vi "Init.vi"(8 "error in (no error)":errorcluster, 11 "Data in":refnum<class "SynchType_DBL.lvclass">) -> (0 "error out":errorcluster, 3 "Data out":refnum<class "SynchType_DBL.lvclass">)   [LabVIEW 2021, in "BT.lvlib" / "SynchType_DBL.lvclass"]
doc: "Abstract Data Classes 2.1.1.12\nTim Streeter - TSA\nCopyright (c) 2024, TSA"
uses:
  SynchType_DBL.lvclass
  SynchType_DBL.lvclass/SynchType_DBL.ctl
  Type.ctl
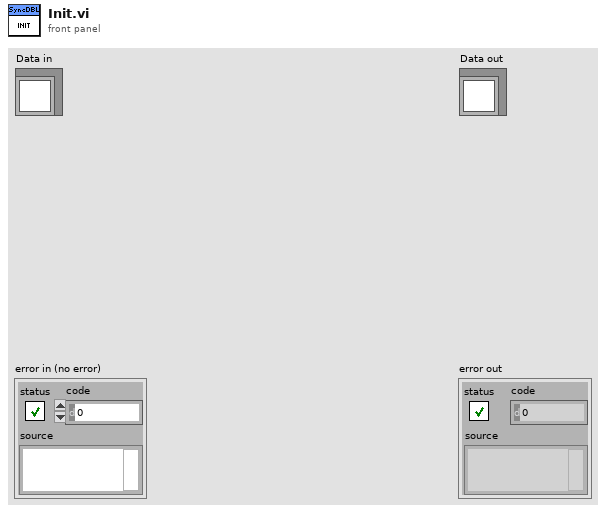
[diagram p1: front panel]
types:
  T1 = typedef "BT.lvlib/SynchType_DBL.lvclass/Type.ctl" = dbl
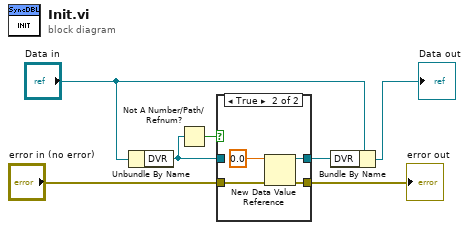
[diagram p0: block diagram]
diagram:
  n1 = Unbundle By Name("Data in") -> ("DVR"=w1:refnum<data-value>)
  n2 = Not A Number/Path/Refnum?(number/path/refnum=w1) -> (NaN/Path/Refnum?=w2:bool)
  n3 = case shown="True" w2 {
    tunnel: "error in (no error)" -> [w8 w13]
    tunnel: [w9 w11] -> w6
    tunnel: [w8 w10] -> w4
    tunnel: w1 -> [w9 _]
    frame False {
    }
    frame True {
      n4 = New Data Value Reference(data value=T1 0.0, error in=w13) -> (data value reference=w11:refnum<data-value>, error out=w10:errorcluster)
    }
  }
  "error out" <- w4
  n5 = Bundle By Name(cluster="Data in", "DVR"=w6) -> (→"Data out":refnum<class "SynchType_DBL.lvclass">)
